vi "Standard table polymorphic.vi"   [LabVIEW 2019, in "Exaprom PDF.lvlib"]
uses:
  Exaprom PDF.lvlib
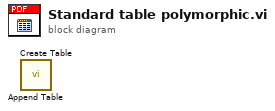
[diagram p0: block diagram]
diagram:
  n1 = call "Append Table.vi"() -> ()  [unwired: 14 in, 2 out]
  n2 = call "Create Table.vi"() -> ()  [unwired: 13 in, 3 out]
